vi "Save intermediate data.vi"(6 "window info":T1={"window type"=3, "window length"=2048} {"window type" items=["None"=0, "Hanning"=1, "Hamming"=2, "Blackman-Harris"=3, "Exact Blackman"=4, "Blackman"=5, "Flat Top"=6, "4 Term B-Harris"=7, "7 Term B-Harris"=8, "Low Sidelobe"=9, "Gaussian"=62]; "window length" min=0}, 7 "prompt":string, 8 "parameters":cluster{"sample rate":sgl, "pulses/rev":i32} {"sample rate" format="%.2f"}, 9 "speed profile":T2 {"speed [RPM]" format="%.2f"; "time [s]" format="%.2f"}, 10 "lables":cluster{"tach lable":string, "S&V lable":string}, 11 "S&V samples":dbl[](array[numeric]) format="%.2f") -> (0 "error out":errorcluster)   [LabVIEW 2017]
uses:
  <vilib>/addons/Sound and Vibration/Order Analysis/Tach Process/SubVIs/speed profile.ctl
  <vilib>/addons/Sound and Vibration/Order Analysis/Ref Gabor Order Tracking/window information.ctl
  <vilib>/addons/Sound and Vibration/Order Analysis/Gabor Order Tracking/SoundVib_Gabor.lvlib
  <vilib>/addons/Sound and Vibration/Order Analysis/Tach Process/SoundVib_TachProcess.lvlib
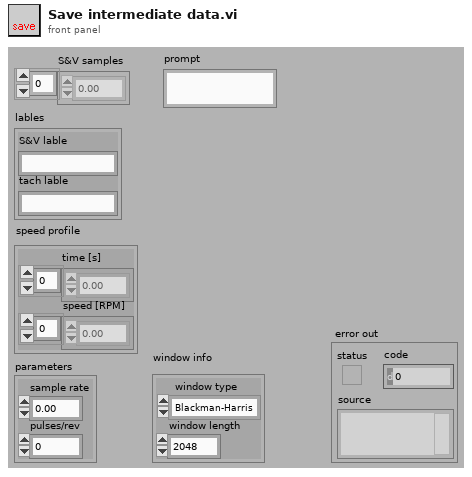
[diagram p1: front panel]
types:
  T1 = typedef "SoundVib_Gabor.lvlib/window information.ctl" = cluster{"window type":u32, "window length":i32}
  T2 = typedef "SoundVib_TachProcess.lvlib/speed profile.ctl" = cluster{"time [s]":dbl[], "speed [RPM]":dbl[]}
  T3 = enum16{"open", "open or create", "create or replace", "create"}
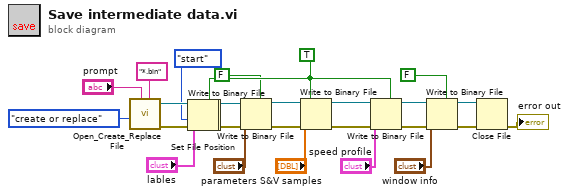
[diagram p0: block diagram]
diagram:
  w5 = TRUE ("header (F)")
  n1 = call <vilib>:"Open_Create_Replace File.vi"("pattern"="*.bin", "prompt"="prompt", "function (open:0)"=T3."create or replace") -> ("error out"=w15:errorcluster, "refnum"=w16:refnum<file>)  [unwired: 5 in, 2 out]
  n2 = Set File Position(refnum=w16, from (0:start)=enum16{"start", "end", "current"}."start" ("pos mode (0:2)"), error in=w15) -> (refnum out=w3:refnum<file>, error out=w2:errorcluster)  [unwired: 1 in]
  n3 = Write to Binary File(file (use dialog)=w3, data="lables", error in=w2, 5:w5) -> (refnum out=w14:refnum<file>, error out=w13:errorcluster)  [unwired: 2 in, 1 out]
  n4 = Write to Binary File(file (use dialog)=w14, data="parameters", error in=w13, 5:FALSE ("prepend array or string size? (T)")) -> (refnum out=w24:refnum<file>, error out=w23:errorcluster)  [unwired: 2 in, 1 out]
  n5 = Write to Binary File(file (use dialog)=w24, data="S&V samples", error in=w23, 5:w5) -> (refnum out=w19:refnum<file>, error out=w18:errorcluster)  [unwired: 2 in, 1 out]
  n6 = Write to Binary File(file (use dialog)=w19, data="speed profile", error in=w18, 5:w5) -> (refnum out=w10:refnum<file>, error out=w9:errorcluster)  [unwired: 2 in, 1 out]
  n7 = Write to Binary File(file (use dialog)=w10, data="window info", error in=w9, 5:FALSE ("prepend array or string size? (T)")) -> (refnum out=w7:refnum<file>, error out=w8:errorcluster)  [unwired: 2 in, 1 out]
  n8 = Close File(refnum=w7, error in=w8) -> (error out=→"error out":errorcluster)  [unwired: 1 out]
